vi "LV SCISDK Read Custom Packet Single Data.vi"(0 "Path":string, 2 "handle":u64, 3 "error in (no error)":errorcluster) -> (7 "function return":i32, 8 "buffer out":T1={"packet_size"=0, "buffer_size"=0, "magic"=0, "valid_data"=0.0, "data"=[10, 100]}, 10 "error out":errorcluster)   [LabVIEW 2021, in "SciSDK_Labview.lvlib"]
doc: "SCISDKLABVIEW_DLL_API int LV_SCISDK_ReadData(char* Path, LV_OSCILLOSCOPE_DECODED_BUFFER* buffer, void* handle);"
uses:
  SciSDK_Labview.lvlib
panel:
  in  "buffer":T2={"magic"=0, "buffer_size"=0, "packet_size"=0, "valid_data"=0, "data"=[10, 100]}
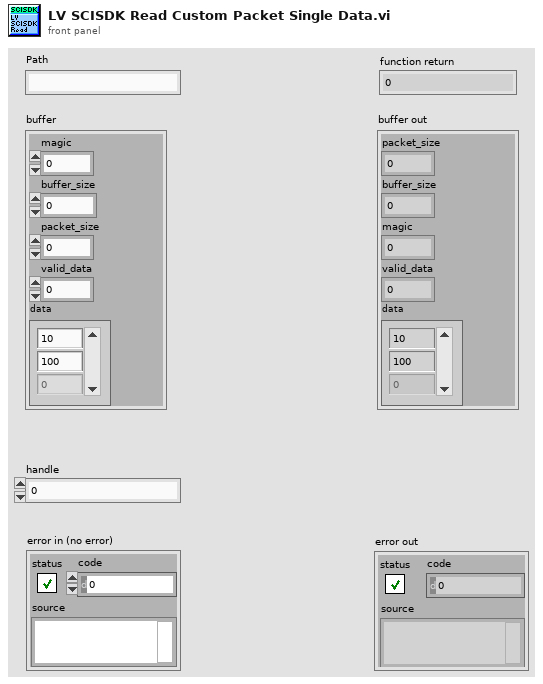
[diagram p1: front panel]
types:
  T1 = cluster{"packet_size":u32, "buffer_size":u32, "magic":u32, "valid_data":dbl, "data":u32[]}
  T2 = cluster{"magic":u32, "buffer_size":u32, "packet_size":u32, "valid_data":u32, "data":u32[]}
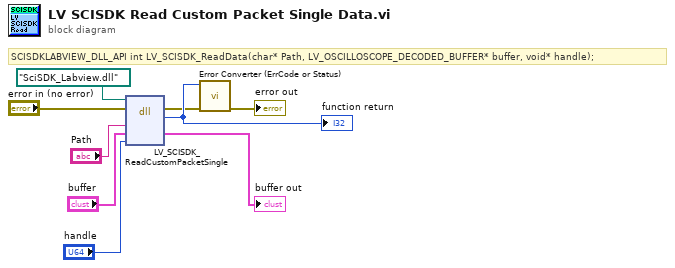
[diagram p0: block diagram]
diagram:
  # "SCISDKLABVIEW_DLL_API int LV_SCISDK_ReadData(char* Path, LV_OSCILLOSCOPE_DECODED_BUFFER* buffer, void* handle);"
  n1 = dll-call lib="C:/git/scisdk/SciSDK_VC++/x64/Debug/SciSDK_Labview.dll" fn="LV_SCISDK_ReadCustomPacketSingle"(path in=path "SciSDK_Labview.dll", error in="error in (no error)", "Path"="Path", "buffer"="buffer", "handle"="handle") -> (error out=w5:errorcluster, "return type"=w9:i32, "buffer"=→"buffer out":T2)  [unwired: 3 in, 1 out]
  "function return" <- w9
  n2 = call <userlib>:"Error Converter (ErrCode or Status).vi"("error in (no error)"=w5, "error code"=w9) -> ("error out"=→"error out":errorcluster)  [unwired: 9 in]
